vi "Set Temperature Set Point.vi"(8 "error in (no error)":errorcluster, 10 "Temperature Set Point":dbl, 11 "Thermal Chamber Controller In":refnum<class "Thermal Chamber Controller.lvclass">) -> (0 "error out":errorcluster, 3 "Thermal Chamber Controller Out":refnum<class "Thermal Chamber Controller.lvclass">)   [LabVIEW 2020, in "Thermal Chamber Controller.lvclass"]
uses:
  Thermal Chamber Controller.lvclass
  <vilib>/Asteme/Triarc Framework/Process/Process.lvclass
  C:/Program Files (x86)/National Instruments/LabVIEW 2020/vi.lib/Asteme/Triarc Framework/View/View.lvclass
  C:/Program Files (x86)/National Instruments/LabVIEW 2020/vi.lib/Asteme/Triarc Framework/Process/Process.lvclass
  C:/Program Files (x86)/National Instruments/LabVIEW 2020/vi.lib/Asteme/Triarc Framework/Base/Base.lvclass
  C:/Program Files (x86)/National Instruments/LabVIEW 2020/vi.lib/Asteme/Triarc Framework/Error Handler Interface/Error Handler Interface.lvclass
  C:/Program Files (x86)/National Instruments/LabVIEW 2020/vi.lib/Asteme/Triarc Framework/Logging/Logging.lvclass
  C:/Users/anton/Documents/GitHub/Triarc-Examples/Thermal Chamber/Thermal Chamber Controller/Thermal Chamber Controller.lvclass
  C:/Program Files (x86)/National Instruments/LabVIEW 2020/vi.lib/Asteme/Triarc Framework/Helper Loop/Helper Loop.lvclass
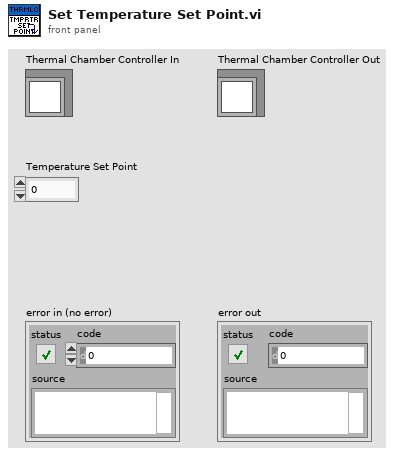
[diagram p1: front panel]
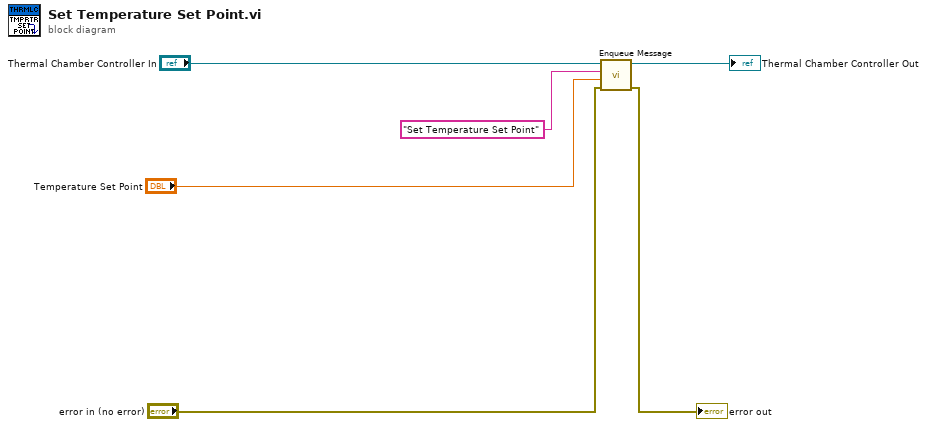
[diagram p0: block diagram]
diagram:
  n1 = call <vilib>:"Enqueue Message.vi"("error in (no error)"="error in (no error)", "Message Data"="Temperature Set Point", "Message"="Set Temperature Set Point" ("API Message"), "Process In"="Thermal Chamber Controller In") -> ("error out"=→"error out":errorcluster, "Process Out"=→"Thermal Chamber Controller Out":refnum<class "Thermal Chamber Controller.lvclass">)  [unwired: 6 in]
